vi "Launch Cryostation UI.vi"() -> ()   [LabVIEW 2016, in "Instrument.Cryostation UI.lvclass"]
doc: "This will launch a stan-alone user interface for the PPMS 2 Instrument\n\nJKI State Machine Objects (SMO) 1.0.0.5\nJKI - JKI\nCopyright (c) 2016, JKI"
uses:
  Instrument.Cryostation UI.lvclass
  <vilib>/JKI/JKI SMO/SMO/SMO.lvclass
  <vilib>/JKI/JKI SMO/SMO.UI/SMO.UI.lvclass
  <vilib>/JKI/JKI SMO/SMO/Typedefs/SMOState --Enum.ctl
  <userlib>/LevyLab/Levylab Instruments/SMOs/Instrument/Typedefs/SMO RC Type--enum.ctl
  <userlib>/LevyLab/Levylab Instruments/SMOs/Instrument/Instrument.lvclass
  <userlib>/LevyLab/Levylab Instruments/SMOs/Instrument/Typedefs/SMO Configuration--Cluster.ctl
  instrument.Cryostation/instrument.Cryostation.lvclass
  <userlib>/LevyLab/Levylab Instruments/SMOs/Instrument UI/Instrument UI.lvclass
  C:/Program Files (x86)/National Instruments/LabVIEW 2016/vi.lib/JKI/JKI SMO/SMO.UI/SMO.UI.lvclass
  C:/Program Files (x86)/National Instruments/LabVIEW 2016/vi.lib/JKI/JKI SMO/SMO/SMO.lvclass
  C:/Program Files (x86)/National Instruments/LabVIEW 2016/user.lib/LevyLab/Levylab Instruments/Instrument Types/Cryostat/Instrument.Cryostat.lvclass
  C:/Program Files (x86)/National Instruments/LabVIEW 2016/user.lib/LevyLab/Levylab Instruments/SMOs/Instrument/Instrument.lvclass
  C:/Program Files (x86)/National Instruments/LabVIEW 2016/user.lib/LevyLab/Levylab Instruments/SMOs/LevyLab/LevyLab.lvclass
panel:
  in  "Address":string
  out "error out":errorcluster
  in  "Stop":bool
  # "Launch Instrument.Cryostation UI UI"
  # "For instructions on how to use the JKI State Machine Objects, examples and video tutorials, visit:\nhttp://jki.net/state-machine-objects/\n\nJKI State Machine Objects™\nhttp://jki.net/state-machine-objects/\nCopyright (C) 2005-2015, JKI <info@jki.net>\nALL RIGHTS RESERVED"
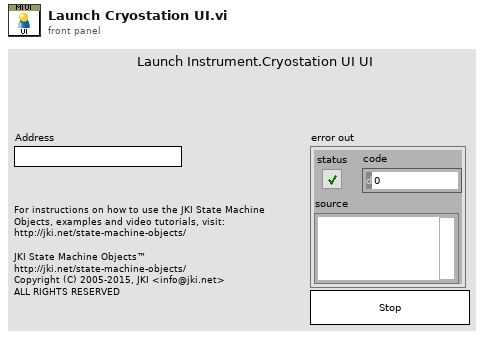
[diagram p1: front panel]
types:
  T1 = typedef "Instrument.lvclass/SMO RC Type--enum.ctl" = enum16{"RC", "STM", "ZMQ"}
  T2 = typedef "Instrument.lvclass/SMO Configuration--Cluster.ctl" = cluster{"Address":string, "Port":u16, "RC Type":T1}
  T3 = typedef "SMO.lvclass/Public Events.ctl" = cluster{"Error":refnum<user-event>, "State":refnum<user-event>, "Reserve State":refnum<user-event>}
  T4 = typedef "SMO.UI.lvclass/PublicEvents--Cluster.ctl" = cluster{"UI Hidden":refnum<user-event>, "UI State":refnum<user-event>}
  T5 = typedef "SMO.lvclass/SMOState --Enum.ctl" = enum16{"unknown", "Created", "Started", "Stopped"}
  T6 = enum32{"Invalid", "Standard", "Closed", "Hidden", "Minimized", "Maximized"}
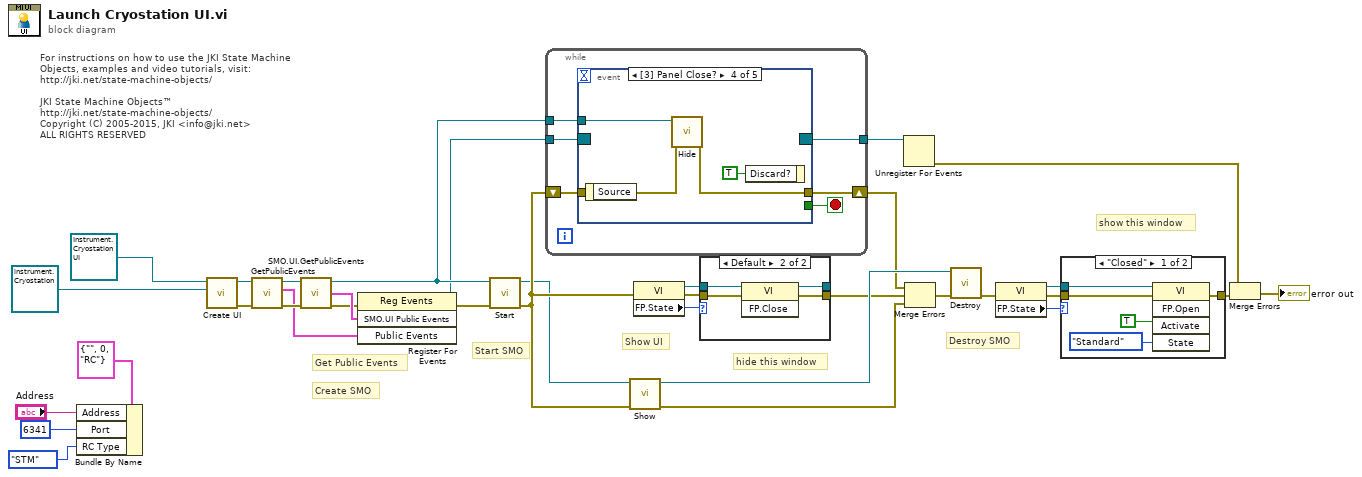
[diagram p0: block diagram]
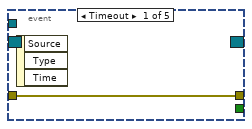
[diagram p4: hidden frame]
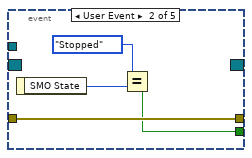
[diagram p5: hidden frame]
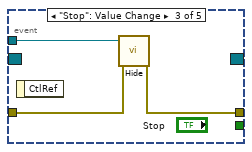
[diagram p6: hidden frame]
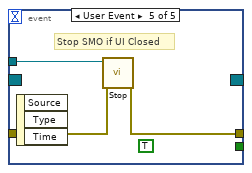
[diagram p7: hidden frame]
diagram:
  # "show this window"
  # "hide this window"
  # "Show UI"
  # "For instructions on how to use the JKI State Machine Objects, examples and video tutorials, visit:\nhttp://jki.net/state-machine-objects/\n\nJKI State Machine Objects™\nhttp://jki.net/state-machine-objects/\nCopyright (C) 2005-2015, JKI <info@jki.net>\nALL RIGHTS RESERVED"
  # "Get Public Events"
  # "Start SMO"
  # "Destroy SMO"
  # "Create SMO"
  n1 = Bundle By Name(cluster=T2 {"Address"="", "Port"=0, "RC Type"=enum."RC"} ("SMO"), "Address"="Address", "Port"=6341, "RC Type"=SMO_RC_Type--enum."STM") -> ()  [unwired: 1 out]
  n2 = call <userlib>:"Create UI.vi"("Instrument in"=refnum<class "instrument.Cryostation.lvclass"> refnum ("instrument.PPMS.lvclass"), "Instrument UI"=refnum<class "Instrument.Cryostation UI.lvclass"> refnum ("SMO.Template.lvclass")) -> ("error out"=w21:errorcluster, "Instrument UI out"=w20:refnum<class "Instrument UI.lvclass">)  [unwired: 8 in]
  n3 = call <vilib>:"GetPublicEvents.vi"("error in (no error)"=w21, "SMO"=w20) -> ("error out"=w23:errorcluster, "Public Events"=w22:T3, "SMO out"=w24:refnum<class "Instrument UI.lvclass">)  [unwired: 7 in]
  n4 = call <vilib>:"SMO.UI.GetPublicEvents.vi"("error in (no error)"=w23, "SMO.UI"=w24) -> ("error out"=w27:errorcluster, "SMO.UI Public Events"=w28:T4, "SMO.UI out"=w29:refnum<class "Instrument UI.lvclass">)  [unwired: 7 in]
  n5 = register-events(error in=w27, w28, w22) -> (reference out=w25:refnum<event-registration>, error out=w26:errorcluster)  [unwired: 1 in]
  n6 = call <vilib>:"Start.vi"("error in (no error)"=w26, "SMO"=w29) -> ("error out"=w17:errorcluster, "SMO out"=w5:refnum<class "Instrument UI.lvclass">)  [unwired: 8 in]
  n7 = while {
    shift-right: [w39] -> w7
    shift-left: w17 -> [w38]
    tunnel: w25 -> [w37]
    tunnel: [w36] -> w34
    tunnel: w29 -> [w35]
    stop <- w40 stop-if-true
    n8 = event shown="[3] Panel Close?" {
      selector: w37 -> [_ _ _ _ _]
      dyn-events: [_ _ _ _ _] -> w36
      timeout: _ -> [_ _ _ _ _]
      tunnel: [_ w42 _ _ _] -> w40
      tunnel: w35 -> [_ _ w48 w51 w55]
      tunnel: [w41 w45 w46 w49 w54] -> w39
      tunnel: w38 -> [w41 w45 w47 w50 w53]
      event Timeout {
        n9 = event-data() -> ()  [unwired: 1 in, 3 out]
      }
      event User Event {
        n10 = event-data() -> ("SMO State"=w44:T5)  [unwired: 1 in]
        n11 = Equal?(x=SMOState_--Enum."Stopped", y=w44) -> (x = y?=w42:bool)
      }
      event "Stop": Value Change {
        n12 = event-data() -> ()  [unwired: 1 in, 1 out]
        n13 = call <vilib>:"Hide.vi"("error in (no error)"=w47, "SMO.UI"=w48) -> ("error out"=w46:errorcluster)  [unwired: 8 in, 1 out]
      }
      event Panel Close? {
        n14 = event-data() -> ()  [unwired: 1 in, 1 out]
        n15 = call <vilib>:"Hide.vi"("error in (no error)"=w50, "SMO.UI"=w51) -> ("error out"=w49:errorcluster)  [unwired: 8 in, 1 out]
        n16 = event-data("Discard?"=TRUE ("OK")) -> ()  [unwired: 1 in, 1 out]
      }
      event User Event {
        (unwired) TRUE ("OK")
        # "Stop SMO if UI Closed"
        n17 = event-data() -> ()  [unwired: 1 in, 3 out]
        n18 = call <vilib>:"Stop.vi"("error in (no error)"=w53, "SMO"=w55) -> ("error out"=w54:errorcluster)  [unwired: 8 in, 1 out]
      }
    }
  }
  n19 = call <vilib>:"Show.vi"("error in (no error)"=w17, "SMO.UI"=w5) -> ("error out"=w6:errorcluster, "SMO.UI out"=w31:refnum<class "Instrument UI.lvclass">)  [unwired: 8 in]
  n20 = property class="VI"(error in=w17) -> (reference out=w15:refnum<vi>, error out=w16:errorcluster, "FP.State"=w14:T6)  [unwired: 1 in]
  n21 = case shown="Default" w14 {
    tunnel: [w57 w61] -> w8
    tunnel: w16 -> [w57 w60]
    tunnel: w15 -> [w56 w59]
    tunnel: [w56 w58] -> _
    frame "Invalid", "Closed" {
    }
    frame Default {
      n22 = invoke class="VI" method="FP.Close"(reference=w59, error in=w60) -> (reference out=w58:refnum<vi>, error out=w61:errorcluster)  [unwired: 1 in, 1 out]
    }
  }
  n23 = Unregister For Events(event registration refnum=w34) -> (error out=w33:errorcluster)  [unwired: 1 in]
  n24 = Merge Errors(w7, w8, w6) -> (w30:errorcluster)
  n25 = call <vilib>:"Destroy.vi"("error in (no error)"=w30, "SMO"=w31) -> ("error out"=w10:errorcluster)  [unwired: 9 in]
  n26 = property class="VI"(error in=w10) -> (reference out=w11:refnum<vi>, error out=w12:errorcluster, "FP.State"=w13:T6)  [unwired: 1 in]
  n27 = case shown="\"Closed\"" w13 {
    tunnel: [w64 w67] -> w9
    tunnel: w12 -> [w63 w67]
    tunnel: w11 -> [w62 _]
    frame "Closed" {
      n28 = invoke class="VI" method="FP.Open"(reference=w62, error in=w63, "Activate"=TRUE, "State"=T6."Standard") -> (error out=w64:errorcluster)  [unwired: 1 in, 4 out]
    }
    frame Default {
    }
  }
  n29 = Merge Errors(w33, w9) -> (→"error out":errorcluster)
